vi "FIR Windowed Filter PtByPt.vi"(0 "x":dbl format="%0.2f", 1 "filter type":T2, 2 "high cutoff freq: fh":dbl=0.45 format="%0.2f", 3 "initialize":bool, 5 "sampling freq: fs":dbl=1.0 format="%0.2f", 9 "window":T1 items=["Rectangle"=0, "Hanning"=1, "Hamming"=2, "Blackman-Harris"=3, "Exact Blackman"=4, "Blackman"=5, "Flat Top"=6, "4 Term B-Harris "=7, "7 Term B-Harris"=8, "Low Sidelobe"=9, "Blackman Nuttall"=11, "Triangle"=30, "Bartlett-Hanning"=31, "Bohman"=32, "Parzen"=33, "Welch"=34, "Kaiser"=60, "Dolph-Chebyshev"=61, "Gaussian"=62], 11 "taps":i32=25, 13 "low cutoff freq: fl":dbl=0.125 format="%0.2f") -> (4 "Filtered x":dbl format="%0.2f", 15 "error":i32)   [LabVIEW 2020, in "NI_PtbyPt.lvlib"]
doc: "Filters <B>x</B> using an FIR filter model."
uses:
  NI_PtbyPt.lvlib
  Filter Passband Type.ctl
  windowTd.ctl
  NI_AALBase.lvlib
  NI_AALPro.lvlib
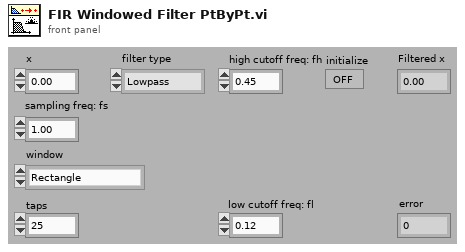
[diagram p1: front panel]
types:
  T1 = typedef "NI_AALPro.lvlib/windowTd.ctl" = u32
  T2 = typedef "NI_AALBase.lvlib/Filter Passband Type.ctl" = enum32{"Lowpass", "Highpass", "Bandpass", "Bandstop"}
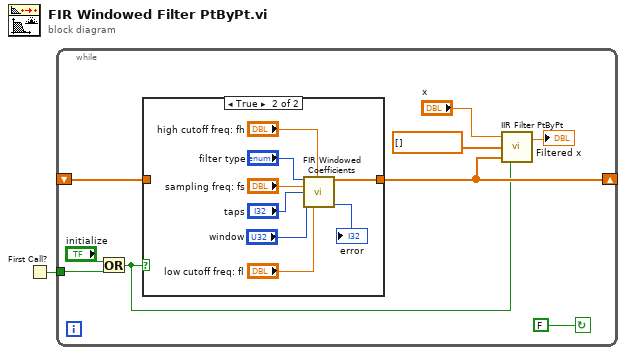
[diagram p0: block diagram]
diagram:
  n1 = First Call?() -> (First Call?: T/F=w1:bool)
  n2 = while {
    tunnel: w1 -> [w2]
    shift-left: _ -> [w7]
    shift-right: [w10] -> _
    stop <- FALSE continue-if-true
    n3 = Or(x="initialize", y=w2) -> (x .or. y?=w3:bool)
    n4 = case shown="True" w3 {
      tunnel: [w11 w19] -> w10
      tunnel: w7 -> [w11 _]
      frame False {
      }
      frame True {
        n5 = call "FIR Windowed Coefficients.vi"("filter type"="filter type", "high cutoff freq: fh"="high cutoff freq: fh", "sampling freq: fs"="sampling freq: fs", "taps"="taps", "window"="window", "low cutoff freq: fl"="low cutoff freq: fl") -> ("FIR Windowed Coefficients"=w19:dbl[], "error"=→"error":i32)  [unwired: 2 in, 6 out]
      }
    }
    n6 = call "IIR Filter PtByPt.vi"("initialize"=w3, "Forward Coefficients"=w10, "Reverse Coefficients"=dbl[] [], "x"="x") -> ("Filtered x"=→"Filtered x":dbl)  [unwired: 1 out]
  }
